vi "Init.vi"(8 "error in (no error)":errorcluster, 9 "Scan Name":string, 10 "Log Path":path, 11 "CSV Test Log in":refnum<class "CSV Test Log.lvclass">) -> (0 "error out":errorcluster, 3 "CSV Test Log out":refnum<class "CSV Test Log.lvclass">)   [LabVIEW 2015, in "CSV Test Log.lvclass"]
uses:
  CSV Test Log.lvclass
  CSV Test Log.lvclass/CSV Test Log.ctl
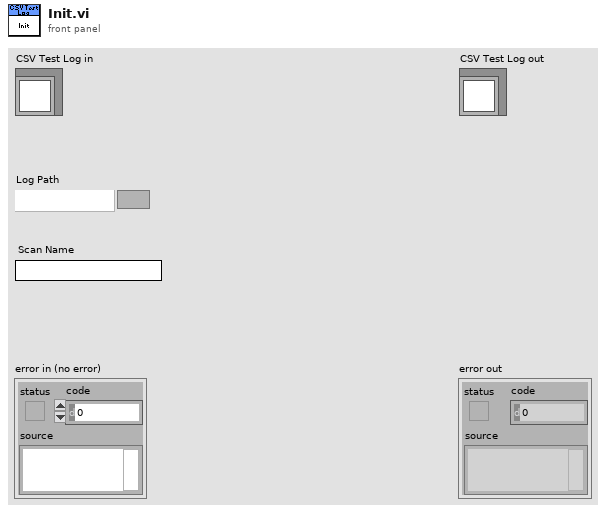
[diagram p1: front panel]
types:
  T1 = enum16{"open", "replace", "create", "open or create", "replace or create", "replace or create with confirmation"}
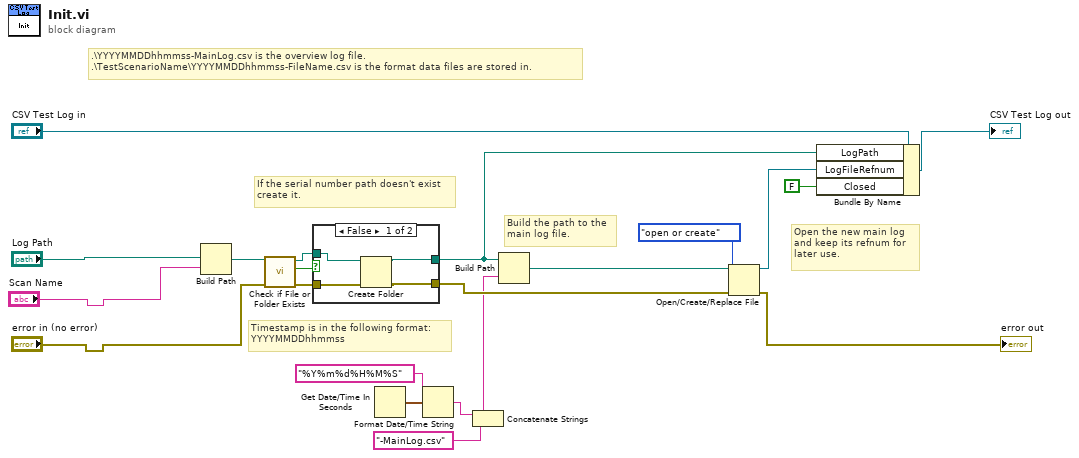
[diagram p0: block diagram]
diagram:
  # "Build the path to the\nmain log file."
  # "Open the new main log\nand keep its refnum for\nlater use."
  # "Timestamp is in the following format:\nYYYYMMDDhhmmss"
  # "If the serial number path doesn't exist\ncreate it."
  # ".\\YYYYMMDDhhmmss-MainLog.csv is the overview log file.\n.\\TestScenarioName\\YYYYMMDDhhmmss-FileName.csv is the format data files are stored in."
  n1 = Build Path(base path="Log Path", name or relative path="Scan Name") -> (appended path=w16:path)
  n2 = call <vilib>:"Check if File or Folder Exists.vi"("error in (no error)"="error in (no error)", "path"=w16) -> ("error out"=w19:errorcluster, "file or folder exists?"=w17:bool, "dup path"=w18:path)  [unwired: 7 in]
  n3 = case shown="False" w17 {
    tunnel: w18 -> [w25 w27]
    tunnel: w19 -> [w24 w26]
    tunnel: [w23 w26] -> w20
    tunnel: [w22 w27] -> w21
    frame False {
      n4 = Create Folder(path (use dialog)=w25, error in=w24) -> (created path=w22:path, error out=w23:errorcluster)  [unwired: 1 in, 1 out]
    }
    frame True {
    }
  }
  n5 = Get Date/Time In Seconds() -> (seconds since 1Jan1904=w11:timestamp)
  n6 = Format Date/Time String(time format string (%c)="%Y%m%d%H%M%S", seconds (now)=w11) -> (date/time string=w13:string)  [unwired: 1 in]
  n7 = Concatenate Strings(w13, "-MainLog.csv" ("string")) -> (w9:string)
  n8 = Build Path(base path=w21, name or relative path=w9) -> (appended path=w14:path)
  n9 = Open/Create/Replace File(file path (use dialog)=w14, error in=w20, operation (0:open)=T1."open or create") -> (refnum out=w15:refnum<file>, error out=→"error out":errorcluster)  [unwired: 3 in, 1 out]
  n10 = Bundle By Name(cluster="CSV Test Log in", "LogPath"=w21, "LogFileRefnum"=w15, "Closed"=FALSE) -> (→"CSV Test Log out":refnum<class "CSV Test Log.lvclass">)
